vi "serialConfigure_p.vi"(2 "genericFlowControl":T1 {"control_char 3" format="%.0x"; "control_char 2" format="%.0x"; "control_char 1" format="%.0x"; "control_char 0" format="%.0x"; "parity error byte" format="%.0x"; "XON byte" format="%.0x"; "XOFF byte" format="%.0x"}, 3 "serialBoard":u16(ring) items=["ttyr", "ttyS"], 4 "serialSettings":T2={"baudRate"=0, "dataBits"=0, "stopBits"=0, "parity"=0, "bufferSize"=8192}, 5 "subID2 (0)":u32, 6 "subID1 (0)":u32, 7 "boardBaseAdd":u32 format="%.0x") -> (0 "errorCode":cdb format="%.2f")   [LabVIEW 2010]
doc: "configures the serial channel (baudrate, handshake and so on...)."
uses:
  <userlib>/libcommon_serial/libcommon_serial.lvlib
panel:
  out "Linux physical device":string
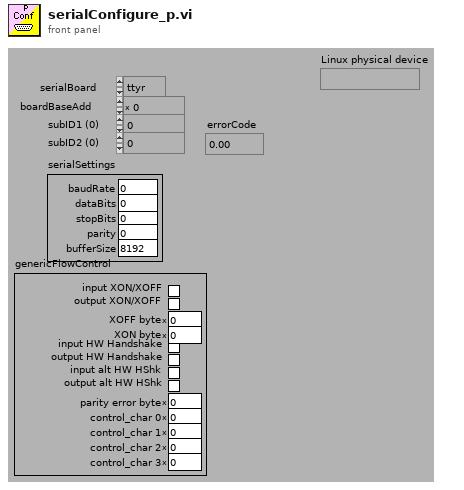
[diagram p1: front panel]
types:
  T1 = cluster{"input XON/XOFF":bool, "output XON/XOFF":bool, "XOFF byte ":u16, "XON byte":u16, "input HW Handshake":bool, "output HW Handshake":bool, "input alt HW HShk":bool, "output alt HW HShk":bool, "parity error byte":u16, "control_char 0":u16, "control_char 1":u16, "control_char 2":u16, "control_char 3":u16}
  T2 = cluster{"baudRate":i32, "dataBits":u16, "stopBits":u16, "parity":u16, "bufferSize":u16}
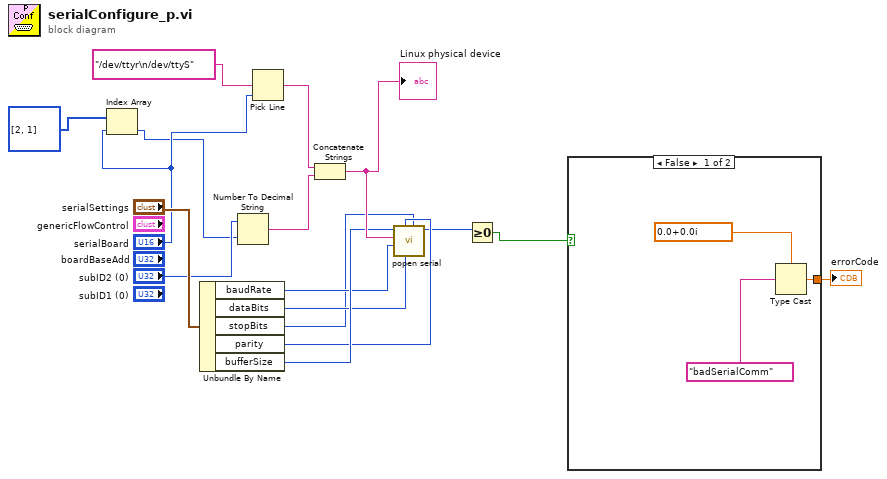
[diagram p0: block diagram]
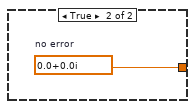
[diagram p2: hidden frame]
diagram:
  n1 = Index Array(array=i16[] [2, 1], index="serialBoard") -> (element=w1:i16)
  n2 = Unbundle By Name("serialSettings") -> ("baudRate"=w11:i32, "dataBits"=w10:u16, "stopBits"=w8:u16, "parity"=w9:u16, "bufferSize"=w12:u16)
  n3 = Number To Decimal String(number="subID2 (0)", width (-)=w1) -> (decimal integer string=w14:string)
  n4 = Pick Line(multi-line string="/dev/ttyr\n/dev/ttyS", line index="serialBoard") -> (output string=w4:string)  [unwired: 1 in]
  n5 = Concatenate Strings(w4, w14) -> (w13:string)
  "Linux physical device" <- w13
  n6 = call <userlib>:"popen serial.vi"("stop"=w8, "bits"=w10, "parity"=w9, "baudrate"=w11, "serdev"=w13, "internal_buffering"=w12) -> ("resourceId"=w6:i32)  [unwired: 4 in, 1 out]
  n7 = Greater Or Equal To 0?(x=w6) -> (x >= 0?=w7:bool)
  n8 = case shown="False" w7 {
    tunnel: [w19 w21] -> w16
    frame False {
      n9 = Type Cast(type=cdb 0.0+0.0i, x="badSerialComm") -> (*(type *) &x=w19:cdb)
    }
    frame True {
      w21 = cdb 0.0+0.0i  # no error
    }
  }
  "errorCode" <- w16
